vi "escrever_ler_dados.vi"() -> ()   [LabVIEW 2018]
uses:
  <vilib>/Instr/_visa.llb/VISA Configure Serial Port (Instr).vi
panel:
  in  "stop":bool
  out "read buffer":string
  in  "String":string
  in  "OK Button":bool
  in  "VISA resource name":refnum<visa-resource-name>
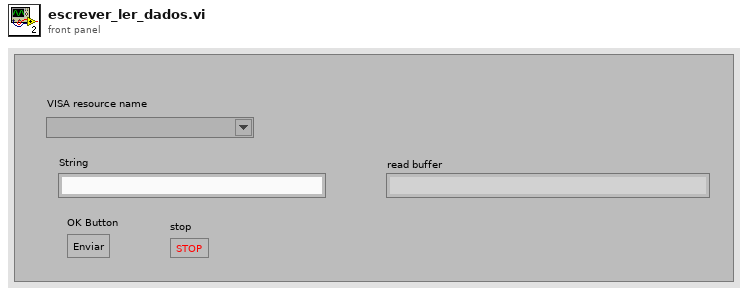
[diagram p1: front panel]
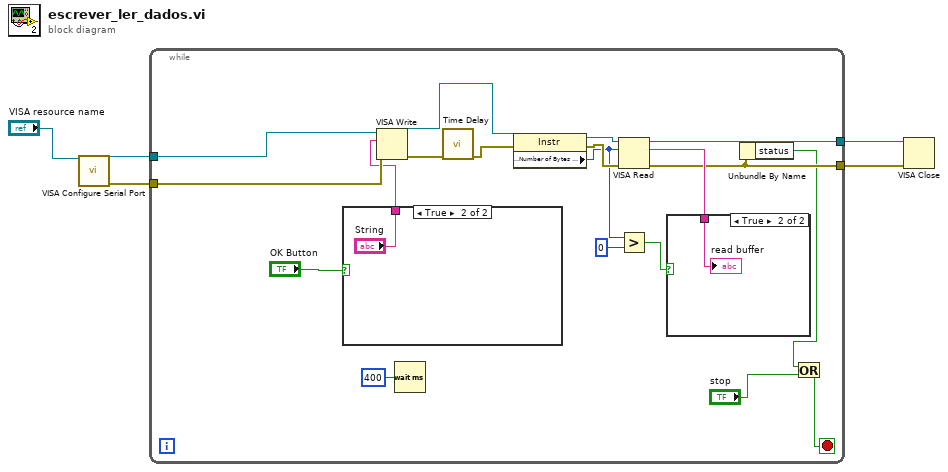
[diagram p0: block diagram]
diagram:
  n1 = call-poly "VISA Configure Serial Port"("VISA resource name"="VISA resource name") -> ("VISA resource name out"=w5:refnum<visa-resource-name>, "error out"=w4:errorcluster)  [unwired: 13 in]
  n2 = while {
    tunnel: w5 -> [w24]
    tunnel: w4 -> [w23]
    tunnel: [w14] -> w2
    tunnel: [w9] -> w1
    stop <- w7 stop-if-true
    n3 = case shown="True" "OK Button" {
      tunnel: [_ "String"] -> w21
      frame False {
      }
      frame True {
      }
    }
    n4 = VISA Write(VISA resource name=w24, write buffer=w21, error in (no error)=w23) -> (VISA resource name out=w16:refnum<visa-resource-name>, error out=w20:errorcluster)  [unwired: 1 out]
    n5 = Wait (ms)(milliseconds to wait=u32 400) -> ()  [unwired: 1 out]
    n6 = call "Time Delay"("error in (no error)"=w20) -> ("error out"=w17:errorcluster)  [unwired: 10 in]
    n7 = property class="Instr"(reference=w16, error in=w17) -> (reference out=w19:refnum<visa-resource-name>, error out=w18:errorcluster, "Serial Settings:Number of Bytes at Serial Port"=w11:u32)
    n8 = VISA Read(VISA resource name=w19, byte count=w11, error in (no error)=w18) -> (VISA resource name out=w14:refnum<visa-resource-name>, read buffer=w13:string, error out=w9:errorcluster)  [unwired: 1 out]
    n9 = Greater?(x=w11, y=u32 0) -> (0:w12:bool)
    n10 = case shown="True" w12 {
      tunnel: w13 -> [_ w25]
      frame False {
      }
      frame True {
        "read buffer" <- w25
      }
    }
    n11 = Unbundle By Name(w9) -> ("status"=w8:bool)
    n12 = Or(x=w8, y="stop") -> (x .or. y?=w7:bool)
  }
  n13 = VISA Close(VISA resource name=w2, error in (no error)=w1) -> ()  [unwired: 1 out]
